vi "PZT_V_LOOP.vi"(8 "间隔":dbl=4.0, 9 "最小电压":dbl=-48.0, 10 "最大电压":dbl=148.0) -> (3 "output array":dbl[](array[numeric]))   [LabVIEW 2019, in "nematic.lvlib"]
uses:
  nematic.lvlib
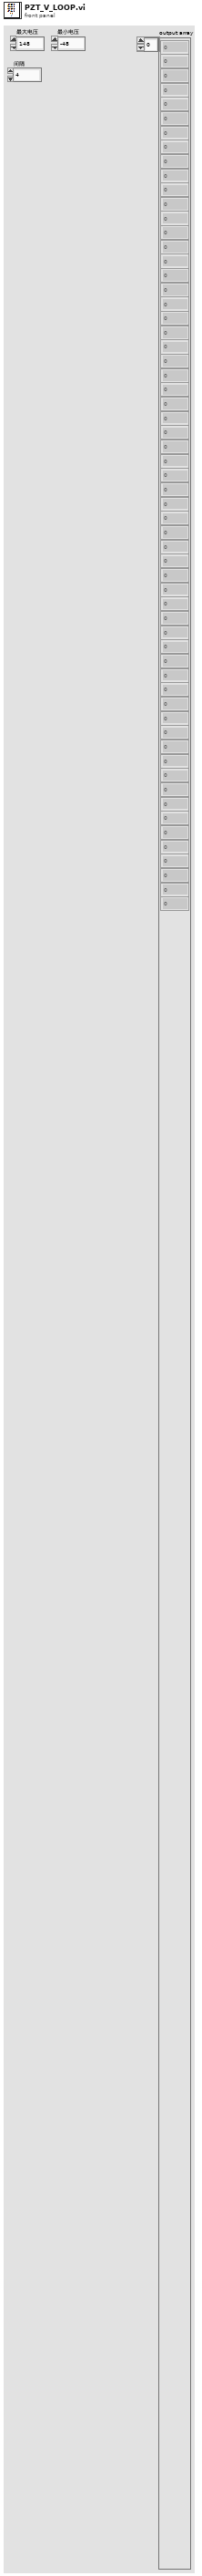
[diagram p1: front panel]
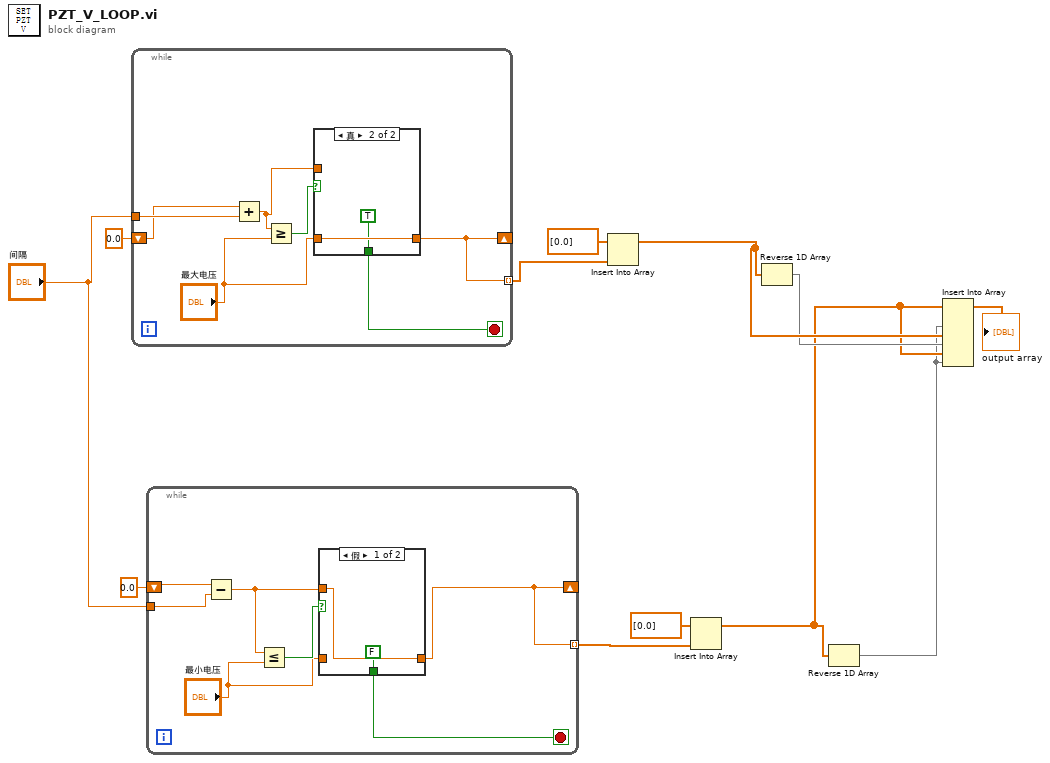
[diagram p0: block diagram]
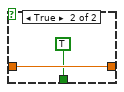
[diagram p2: hidden frame]
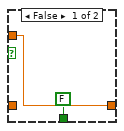
[diagram p3: hidden frame]
diagram:
  n1 = while {
    tunnel: "间隔" -> [w19]
    shift-right: [w13] -> _
    shift-left: 0.0 ("最大电压") -> [w16]
    tunnel: [w13] -> w8 mode=indexing
    stop <- w15 stop-if-true
    n2 = Add(x=w16, y=w19) -> (x+y=w14:dbl)
    n3 = Greater Or Equal?(x=w14, y="最大电压") -> (x >= y?=w18:bool)
    n4 = case shown="真" w18 {
      tunnel: "最大电压" -> [_ w23]
      tunnel: [w21 w23] -> w13
      tunnel: [FALSE TRUE] -> w15
      tunnel: w14 -> [w21 _]
      frame False {
      }
      frame True {
      }
    }
  }
  n5 = while {
    shift-right: [w24] -> _
    shift-left: 0.0 -> [w30]
    tunnel: "间隔" -> [w29]
    tunnel: [w24] -> w6 mode=indexing
    stop <- w26 stop-if-true
    n6 = Subtract(x=w30, y=w29) -> (x-y=w28:dbl)
    n7 = Less Or Equal?(x=w28, y="最小电压") -> (x <= y?=w27:bool)
    n8 = case shown="假" w27 {
      tunnel: "最小电压" -> [_ w34]
      tunnel: [w32 w34] -> w24
      tunnel: [FALSE TRUE] -> w26
      tunnel: w28 -> [w32 _]
      frame False {
      }
      frame True {
      }
    }
  }
  n9 = Insert Into Array(array=dbl[] [0.0], new element=w8) -> (w5:dbl[])  [unwired: 1 in]
  n10 = Insert Into Array(array=dbl[] [0.0], new element=w6) -> (w3:dbl[])  [unwired: 1 in]
  n11 = Reverse 1D Array(array=w5) -> (reversed array=w4:dbl[])
  n12 = Reverse 1D Array(array=w3) -> (reversed array=w2:dbl[])
  n13 = Insert Into Array(array=w3, new element #1=w2, new element #2=w5, new element #3=w4, new element #4=w3, new element #5=w2) -> (→"output array":dbl[])  [unwired: 1 in]
